vi "Set Default Value.vi"(9 "Default C++ Value":string, 10 "Control Ref":refnum<vi>, 11 "Bool Writer in":refnum<class "Bool Writer.lvclass">) -> (1 "LabVIEW Default String":string, 2 "Control Ref Dup":refnum<vi>, 3 "Bool Writer out":refnum<class "Bool Writer.lvclass">)   [LabVIEW 2014, in "Bool Writer.lvclass"]
doc: "Copyright (c) 2016 Sze Howe Koh\n\nThis Source Code Form is subject to the terms of the Mozilla Public License, v. 2.0. If a copy of the MPL was not distributed with this file, You can obtain one at http://mozilla.org/MPL/2.0/."
uses:
  Bool Writer.lvclass
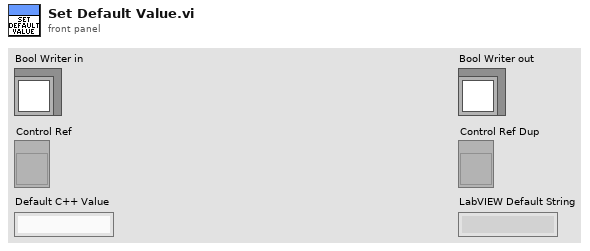
[diagram p1: front panel]
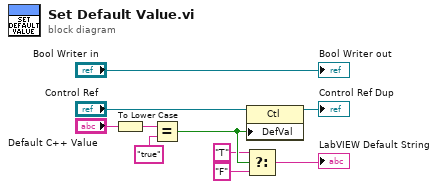
[diagram p0: block diagram]
diagram:
  n1 = To Lower Case(string="Default C++ Value") -> (all lower case string=w7:string)
  n2 = Equal?(x=w7, y="true") -> (x = y?=w5:bool)
  n3 = property class="Ctl"(reference="Control Ref", "DefVal"=w5) -> (reference out=→"Control Ref Dup":refnum<vi>)  [unwired: 1 in, 1 out]
  n4 = Select(t="T" ("y"), s=w5, f="F" ("y")) -> (s? t:f=→"LabVIEW Default String":string)
  "Bool Writer out" <- "Bool Writer in"
